vi "GetAllFolderContents.vi"(11 "Path":path) -> (3 "Folder Listings":T1[](array[typedef]))   [LabVIEW 2024]
uses:
  TypeDefs/FolderContents.ctl
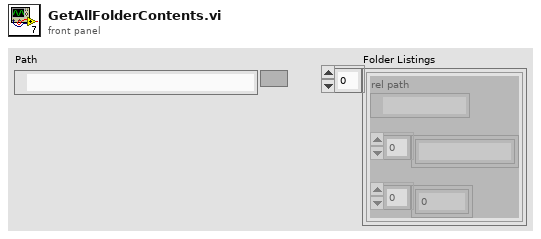
[diagram p1: front panel]
types:
  T1 = typedef "FolderContents.ctl" = cluster{"rel path":path, "file names":string[], "file sizes":i64[]}
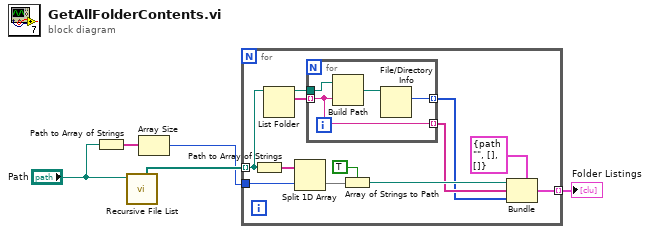
[diagram p0: block diagram]
diagram:
  n1 = Path to Array of Strings(0:"Path") -> (2:w4:string[])  [unwired: 1 out]
  n2 = call <vilib>:"Recursive File List.vi"("Folder Path"="Path") -> ("All Folders"=w3:path[])  [unwired: 6 in, 4 out]
  n3 = Array Size(array=w4) -> (size(s)=w2:i32)
  n4 = for {
    tunnel: w3 -> [w13] mode=indexing
    tunnel: w2 -> [w16]
    tunnel: [w10] -> w1 mode=indexing
    n5 = Path to Array of Strings(0:w13) -> (2:w17:string[])  [unwired: 1 out]
    n6 = List Folder(path=w13) -> (path out=w11:path, filenames=w12:string[])  [unwired: 3 in, 2 out]
    n7 = Split 1D Array(array=w17, index=w16) -> (second subarray=w15:string[])  [unwired: 1 out]
    n8 = for {
      tunnel: w12 -> [w19] mode=indexing
      tunnel: w11 -> [w21]
      tunnel: [w19] -> w8 mode=indexing
      tunnel: [w18] -> w7 mode=indexing
      n9 = Build Path(base path=w21, name or relative path=w19) -> (appended path=w20:path)
      n10 = File/Directory Info(path=w20) -> (size=w18:i64)  [unwired: 1 in, 6 out]
    }
    n11 = Array of Strings to Path(0:w15, 1:TRUE ("relative")) -> (2:w9:path)
    n12 = Bundle(cluster=T1 {"rel path"=path "", "file names"=[], "file sizes"=[]} ("FolderContents"), "rel path"=w9, "file names"=w8, "file sizes"=w7) -> (w10:T1)
  }
  "Folder Listings" <- w1
